vi "AnalyzeDeviationMeasurement.vi"(8 "Peak detected?":bool, 9 "Gauss residue control reference in":refnum<vi>, 10 "Graph control reference in":refnum<vi>, 11 "Measured data":cluster{dbl[], dbl[]}) -> (0 "Gauss center position [mm]":dbl, 1 "Gauss residue control reference out":refnum<vi>, 2 "Graph control reference out":refnum<vi>)   [LabVIEW 2013]
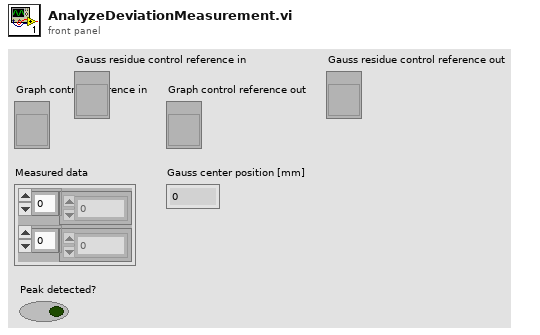
[diagram p1: front panel]
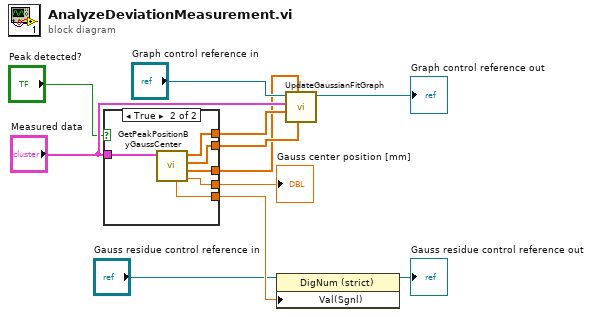
[diagram p0: block diagram]
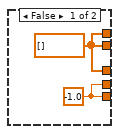
[diagram p2: hidden frame]
diagram:
  n1 = case shown="True" "Peak detected?" {
    tunnel: "Measured data" -> [_ w19]
    tunnel: [w12 w18] -> w4
    tunnel: [w13 w17] -> w6
    tunnel: [w13 w16] -> w10
    tunnel: [w13 w15] -> w11
    tunnel: [w12 w14] -> w3
    frame False {
      w13 = dbl[] [] ("Peak amplitudes")
      w12 = -1.0 ("Peak position [mm]")
    }
    frame True {
      n2 = call "GetPeakPositionByGaussCenter.vi"("Input cluster"=w19) -> ("Gauss center position [mm]"=w18:dbl, "Best Gaussian Fit"=w17:dbl[], "Peak amplitudes"=w15:dbl[], "Peak locations"=w16:dbl[], "Gauss residue"=w14:dbl)  [unwired: 6 in]
    }
  }
  "Gauss center position [mm]" <- w4
  n3 = property class="DigNum (strict)"(reference="Gauss residue control reference in", "Val(Sgnl)"=w3) -> (reference out=→"Gauss residue control reference out":refnum<vi>)  [unwired: 1 in, 1 out]
  n4 = call "UpdateGaussianFitGraph.vi"("Peak amplitudes"=w11, "Best Gaussian Fit"=w6, "Peak locations"=w10, "Original measured data"="Measured data", "Control in"="Graph control reference in") -> ("Control out"=→"Graph control reference out":refnum<vi>)  [unwired: 6 in]
